vi "Test Objekt Referenzen.vi"() -> ()   [LabVIEW 2020]
uses:
  Steuerung PNS.lvclass
panel:
  out "IP Adresse":string="192.168.15.101"
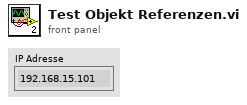
[diagram p1: front panel]
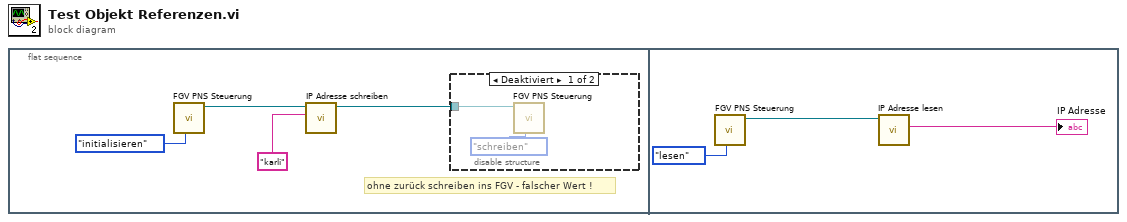
[diagram p0: block diagram]
diagram:
  n1 = flat-sequence {
    frame #0 {
      # "ohne zurück schreiben ins FGV - falscher Wert !"
      n2 = call "FGV PNS Steuerung.vi"("Enum"=enum16{"initialisieren", "lesen", "schreiben"}."initialisieren") -> ("Steuerung PNS (Ausgang)"=w3:refnum<class "Steuerung PNS.lvclass">)  [unwired: 10 in]
      n3 = call-dynamic "IP Adresse schreiben.vi"("IP Adresse"="karli" ("IP-Adresse"), "Steuerung PNS (Eingang)"=w3) -> ("Steuerung PNS (Ausgang)"=w1:refnum<class "Steuerung PNS.lvclass">)  [unwired: 8 in, 1 out]
      n4 = disable-structure shown="Deaktiviert" {
        disable-tunnel: w1 -> [w6 _]
        frame Disabled {
          n5 = call "FGV PNS Steuerung.vi"("Enum"=enum16{"initialisieren", "lesen", "schreiben"}."schreiben", "Steuerung PNS (Eingang)"=w6) -> ()  [unwired: 9 in, 1 out]
        }
        frame Enabled {
        }
      }
    }
    frame #1 {
      n6 = call "FGV PNS Steuerung.vi"("Enum"=enum16{"initialisieren", "lesen", "schreiben"}."lesen") -> ("Steuerung PNS (Ausgang)"=w8:refnum<class "Steuerung PNS.lvclass">)  [unwired: 10 in]
      n7 = call-dynamic "IP Adresse lesen.vi"("Steuerung PNS (Eingang)"=w8) -> ("IP Adresse"=→"IP Adresse":string)  [unwired: 8 in, 2 out]
    }
  }
